vi "visuallyInspectPositionListResults.vi"() -> ()   [LabVIEW 2016]
uses:
  <vilib>/vision/driver/NI_Vision_Acquisition_Software.lvlib
  <vilib>/vision/NI_Vision_Development_Module.lvlib
  <vilib>/regexp/Match Regular Expression.xnode
  <vilib>/Utility/file.llb/Write Delimited Spreadsheet (DBL).vi
panel:
  in  "Gain":dbl(slide)=4.875739644970414 scale=0.0..20.0
  in  "Nloops":i32=1
  in  "OK Button - Dump":bool
  in  "Path to save collected images":path=path "E:/BNL/XYZstage+Camera_CollectedImages/01-31-2017/Images"
  in  "OK Button - Save":bool
  out "Finished!":bool
  out "Image #":i32=79
  out "Error report":errorcluster
  out "Most recently collected image":T1(plugin-control)
  out "XYZ Stage Current Position":T2={"X [-750, 750 mm]"=-61.75289519379574, "Y [-150, 30 mm]"=-124.53559346701012, "Z [-50, 50 mm]"=-0.8115271662620002}
  in  "Axes Speeds [mm/s]":T3={"X Speed"=25.0, "Y Speed"=10.0, "Z Speed"=10.0}
  out "Moving":bool
  in  "Camera Name":refnum<k21>="cam0" caption="IMAQdx Session"
  in  "Object Location [mm]":T4={"Go to X"=-61.753, "Go to Y"=-124.535, "Go to Z"=-0.811426}
  in  "error in (no error)":errorcluster
  in  "Set of Coordinates to Process":dbl[][](array[numeric])=[[-61.665, -28.54, 0.0], [-61.66, -29.04, -0.05], [35.36, -28.5689, -0.5], [35.359, -29.07, -0.5], [35.35, -125.048, -1.1309], [35.327, -124.561, -1.165], [-61.7, -125.017, -0.8146], [-61.753, -124.535, -0.811426], [-61.665, -28.54, 0.0], [-61.66, -29.04, -0.05], [35.36, -28.5689, -0.5], [35.359, -29.07, -0.5], [35.35, -125.048, -1.1309], [35.327, -124.561, -1.165], [-61.7, -125.017, -0.8146], [-61.753, -124.535, -0.811426], [-61.665, -28.54, 0.0], [-61.66, -29.04, -0.05], [35.36, -28.5689, -0.5], [35.359, -29.07, -0.5], [35.35, -125.048, -1.1309], [35.327, -124.561, -1.165], [-61.7, -125.017, -0.8146], [-61.753, -124.535, -0.811426], [-61.665, -28.54, 0.0], [-61.66, -29.04, -0.05], [35.36, -28.5689, -0.5], [35.359, -29.07, -0.5], [35.35, -125.048, -1.1309], [35.327, -124.561, -1.165], [-61.7, -125.017, -0.8146], [-61.753, -124.535, -0.811426], [-61.665, -28.54, 0.0], [-61.66, -29.04, -0.05], [35.36, -28.5689, -0.5], [35.359, -29.07, -0.5], [35.35, -125.048, -1.1309], [35.327, -124.561, -1.165], [-61.7, -125.017, -0.8146], [-61.753, -124.535, -0.811426], [-61.665, -28.54, 0.0], [-61.66, -29.04, -0.05], [35.36, -28.5689, -0.5], [35.359, -29.07, -0.5], [35.35, -125.048, -1.1309], [35.327, -124.561, -1.165], [-61.7, -125.017, -0.8146], [-61.753, -124.535, -0.811426], [-61.665, -28.54, 0.0], [-61.66, -29.04, -0.05], [35.36, -28.5689, -0.5], [35.359, -29.07, -0.5], [35.35, -125.048, -1.1309], [35.327, -124.561, -1.165], [-61.7, -125.017, -0.8146], [-61.753, -124.535, -0.811426], [-61.665, -28.54, 0.0], [-61.66, -29.04, -0.05], [35.36, -28.5689, -0.5], [35.359, -29.07, -0.5], [35.35, -125.048, -1.1309], [35.327, -124.561, -1.165], [-61.7, -125.017, -0.8146], [-61.753, -124.535, -0.811426], [-61.665, -28.54, 0.0], [-61.66, -29.04, -0.05], [35.36, -28.5689, -0.5], [35.359, -29.07, -0.5], [35.35, -125.048, -1.1309], [35.327, -124.561, -1.165], [-61.7, -125.017, -0.8146], [-61.753, -124.535, -0.811426], [-61.665, -28.54, 0.0], [-61.66, -29.04, -0.05], [35.36, -28.5689, -0.5], [35.359, -29.07, -0.5], [35.35, -125.048, -1.1309], [35.327, -124.561, -1.165], [-61.7, -125.017, -0.8146], [-61.753, -124.535, -0.811426]]
  out "Image Array":T1[](array[plugin-control])
  # "Use the index box to specify the image you wish to view"
  # ">>>>"
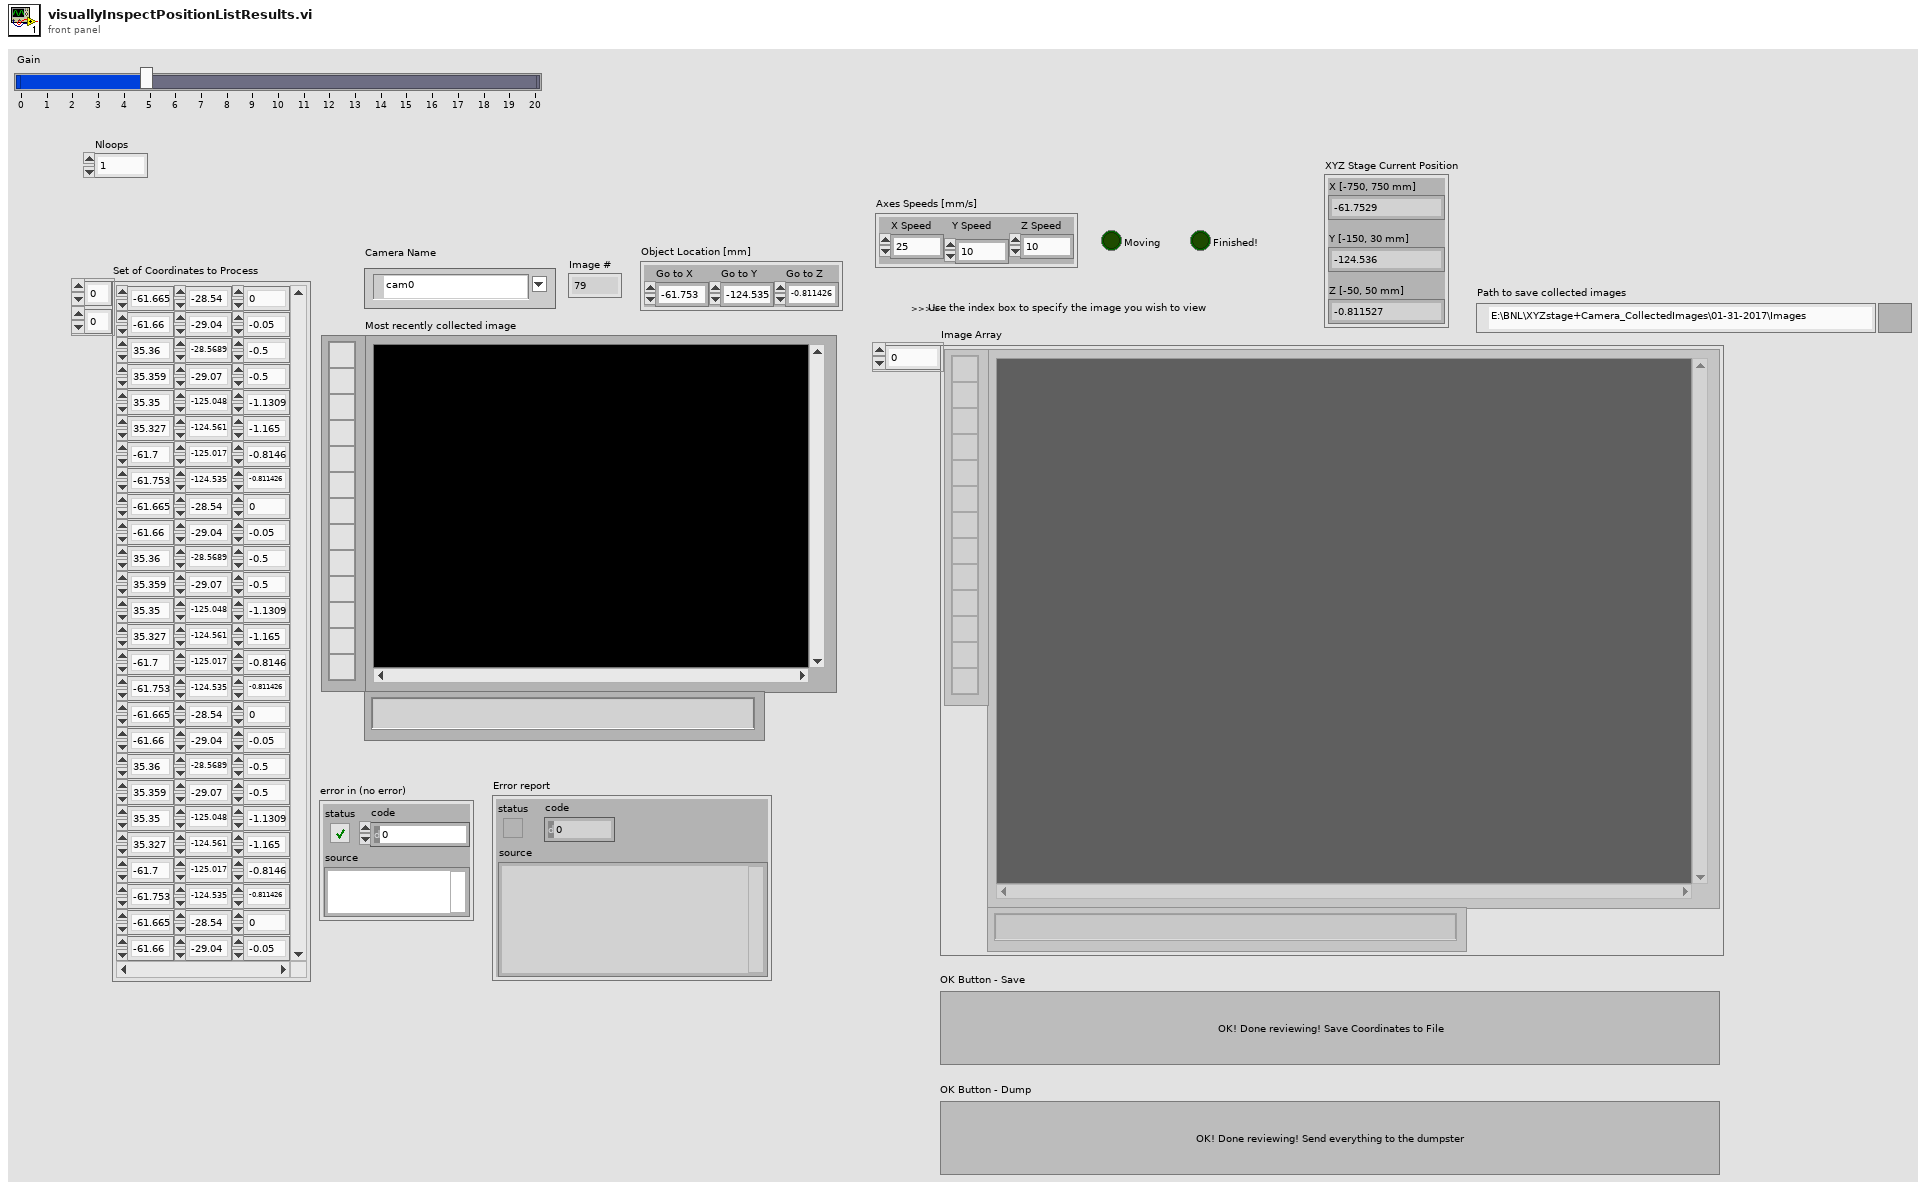
[diagram p1: front panel]
types:
  T1 = typedef "IMAQ Image.ctl" = refnum<image>
  T2 = cluster{"X [-750, 750 mm]":dbl, "Y [-150, 30 mm]":dbl, "Z [-50, 50 mm]":dbl}
  T3 = cluster{"X Speed":dbl, "Y Speed":dbl, "Z Speed":dbl}
  T4 = cluster{"Go to X":dbl, "Go to Y":dbl, "Go to Z":dbl}
  T5 = typedef "IMAQdx.ctl" = refnum<k21>
  T6 = cluster{"Set of Coordinates to Process[0]":dbl, "Set of Coordinates to Process[1]":dbl, "Set of Coordinates to Process[2]":dbl}
  T7 = typedef "Image Type" = u32
  T8 = cluster{"Final X":dbl, "Final Y":dbl, "Final Z":dbl}
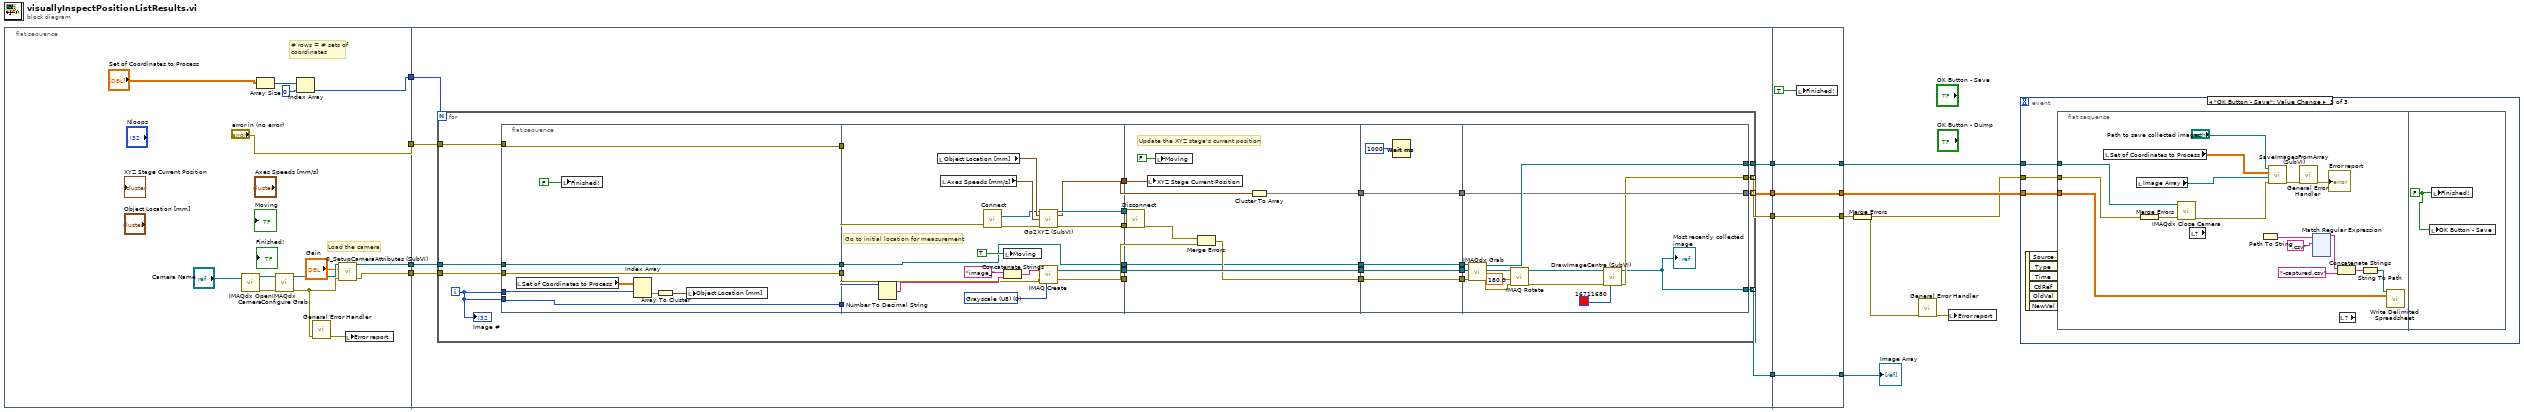
[diagram p0: block diagram]
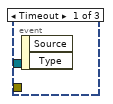
[diagram p2: hidden frame]
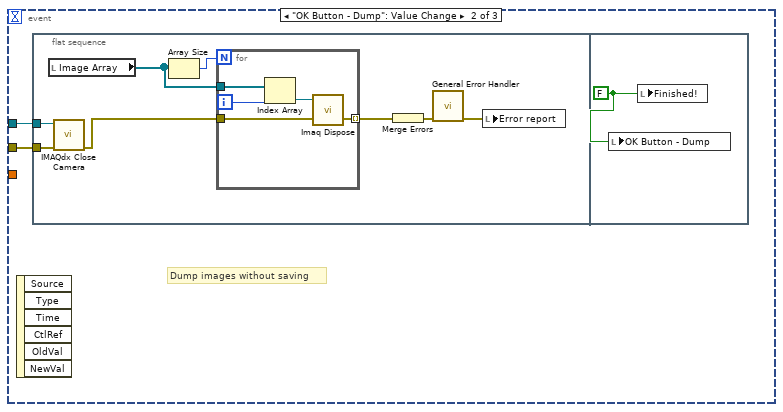
[diagram p3: hidden frame]
diagram:
  n1 = flat-sequence {
    tunnel: [w25] -> w4
    tunnel: ["error in (no error)"] -> w3
    tunnel: [w16] -> w2
    tunnel: [w15] -> w1
    tunnel: [w35] -> w8
    tunnel: [w34] -> w7
    tunnel: [w33] -> w6
    tunnel: [w31] -> w5
    tunnel: w4 -> [w36]
    tunnel: w3 -> [w32]
    tunnel: w2 -> [w30]
    tunnel: w1 -> [w29]
    tunnel: [w119] -> w11
    tunnel: [w120] -> w12
    tunnel: [w121] -> w13
    tunnel: [w122] -> w14
    tunnel: w8 -> [w122]
    tunnel: w7 -> [w121]
    tunnel: w6 -> [w120]
    tunnel: w5 -> [w119]
    frame #0 {
      # "Load the camera"
      # "# rows = # sets of\ncoordinates"
      n2 = call <vilib>:"IMAQdx Open Camera.vi"("Session In"="Camera Name") -> ("error out"=w18:errorcluster, "Session Out"=w17:T5)  [unwired: 2 in, 7 out]
      n3 = Array Size(array="Set of Coordinates to Process") -> (size(s)=w26:i32[])
      n4 = call <vilib>:"IMAQdx Configure Grab.vi"("error in"=w18, "Session In"=w17) -> ("error out"=w22:errorcluster, "Session Out"=w23:T5)  [unwired: 8 out]
      n5 = Index Array(array=w26, index=0) -> (element=w25:i32)
      n6 = call <vilib>:"General Error Handler.vi"("error in (no error)"=w22) -> ("error out"=w20:errorcluster)  [unwired: 2 in, 12 out]
      n7 = call "0_SetupCameraAttributes (SubVI).vi"("error in (no error)"=w22, "Gain"="Gain", "Camera session in"=w23) -> ("error out"=w16:errorcluster, "Camera session out"=w15:T5)  [unwired: 7 in]
      n8 = local write "Error report"(w20) -> ()
    }
    frame #1 {
      n9 = for {
        N: w36 -> [_]
        tunnel: [w54] -> w35 mode=indexing
        tunnel: w32 -> [w52]
        tunnel: w30 -> [w50]
        tunnel: [w46] -> w34
        tunnel: [w45] -> w31 mode=indexing
        tunnel: [w42] -> w33 mode=indexing
        tunnel: w29 -> [w41]
        i -> [w58]
        n10 = flat-sequence {
          tunnel: w58 -> [w68]
          tunnel: w58 -> [w67]
          tunnel: [w67] -> w59
          tunnel: [w66] -> w53
          tunnel: w52 -> [w66]
          tunnel: [w65] -> w51
          tunnel: w50 -> [w65]
          tunnel: w41 -> [w63]
          tunnel: [w63] -> w40
          tunnel: [w83] -> w62
          tunnel: [w82] -> w61
          tunnel: [w81] -> w60
          tunnel: w59 -> [w77]
          tunnel: [w78] -> w55
          tunnel: w53 -> [w75]
          tunnel: w51 -> [w74]
          tunnel: [w73] -> w47
          tunnel: w40 -> [w72]
          tunnel: [w72] -> w39
          tunnel: w62 -> [w98]
          tunnel: w61 -> [w92]
          tunnel: w60 -> [w97]
          tunnel: [w96] -> w56
          tunnel: w55 -> [w96]
          tunnel: [w93] -> w48
          tunnel: w47 -> [w94]
          tunnel: [w91] -> w44
          tunnel: w39 -> [w90]
          tunnel: [w90] -> w37
          tunnel: [w103] -> w57
          tunnel: w56 -> [w103]
          tunnel: [w102] -> w49
          tunnel: w48 -> [w102]
          tunnel: w44 -> [w101]
          tunnel: [w101] -> w43
          tunnel: [w100] -> w38
          tunnel: w37 -> [w100]
          tunnel: w57 -> [w117]
          tunnel: [w107] -> w54
          tunnel: w49 -> [w114]
          tunnel: [w112] -> w46
          tunnel: [w108] -> w45
          tunnel: w43 -> [w111]
          tunnel: [w111] -> w42
          tunnel: w38 -> [w105]
          frame #0 {
            n11 = local read "Set of Coordinates to Process"() -> (w69:dbl[][])
            n12 = local write "Finished!"(FALSE ("Finished!")) -> ()
            n13 = Index Array(array=w69, index (row)=w68) -> (element=w70:dbl[])  [unwired: 1 in]
            n14 = Array To Cluster(array=w70) -> (cluster=w71:T6)
            n15 = local write "Object Location [mm]"(w71) -> ()
          }
          frame #1 {
            w89 = T7 0 items=["Grayscale (U8)", "Grayscale (I16)", "Grayscale (SGL)", "Complex (CSG)", "RGB (U32)", "HSL (U32)", "RGB (U64)", "Grayscale (U16)"] ("Image Type")
            # "Go to initial location for measurement"
            n16 = Number To Decimal String(number=w77) -> (decimal integer string=w76:string)  [unwired: 1 in]
            n17 = local read "Object Location [mm]"() -> (w86:T4)
            n18 = local read "Axes Speeds [mm/s]"() -> (w87:T3)
            n19 = call "Connect.vi"("error in (no error)"=w75) -> ("error out"=w84:errorcluster, "controller"=w85:refnum<k24>)  [unwired: 9 in]
            n20 = local write "Moving"(TRUE ("Moving")) -> ()
            n21 = Concatenate Strings("image_" ("Image Name"), w76) -> (w79:string)
            n22 = call "Go2XYZ (SubVI).vi"(".NET Refnum in"=w85, "Go to Coordinates"=w86, "Axis Speeds"=w87, "error in (no error)"=w84) -> (".NET Refnum out"=w83:refnum<k24>, "Final Position"=w82:T8, "error out"=w81:errorcluster)  [unwired: 7 in, 2 out]
            n23 = call "IMAQ Create"("Image Name"=w79, "Image Type"=w89, "error in (no error)"=w74) -> ("New Image"=w78:T1, "error out"=w73:errorcluster)  [unwired: 1 in, 1 out]
          }
          frame #2 {
            # "Update the XYZ stage's current position"
            n24 = call "Disconnect.vi"("error in (no error)"=w97, "controller"=w98) -> ("error out"=w95:errorcluster)  [unwired: 9 in]
            n25 = local write "XYZ Stage Current Position"(w92) -> ()
            n26 = local write "Moving"(FALSE ("Moving")) -> ()
            n27 = Merge Errors(w95, w94) -> (w93:errorcluster)
            n28 = Cluster To Array(cluster=w92) -> (array=w91:dbl[])
          }
          frame #3 {
            n29 = Wait (ms)(milliseconds to wait=u32 1000) -> ()  [unwired: 1 out]
          }
          frame #4 {
            n30 = call <vilib>:"IMAQdx Grab.vi"("error in"=w114, "Image In"=w117, "Session In"=w105) -> ("error out"=w113:errorcluster, "Image Out"=w116:T1, "Session Out"=w112:T5)  [unwired: 1 in, 5 out]
            n31 = call "IMAQ Rotate"("error in (no error)"=w113, "Angle (degrees)"=sgl 180.0, "Image Src"=w116) -> ("error out"=w109:errorcluster, "Image Dst Out"=w110:T1)  [unwired: 7 in]
            n32 = call "DrawImageCentre (SubVI).vi"("Axis colour"=u32 16711680, "error in (no error)"=w109, "Refnum in"=w110) -> ("error out"=w108:errorcluster, "Refnum out"=w107:T1)  [unwired: 7 in]
            "Most recently collected image" <- w107
          }
        }
        "Image #" <- w58
      }
    }
    frame #2 {
      n33 = local write "Finished!"(TRUE ("Finished!")) -> ()
    }
  }
  n34 = Merge Errors(w11) -> (w9:errorcluster)
  n35 = call <vilib>:"General Error Handler.vi"("error in (no error)"=w9) -> ("error out"=w10:errorcluster)  [unwired: 2 in, 12 out]
  n36 = local write "Error report"(w10) -> ()
  n37 = event shown="[2] \"OK Button - Save\": Value Change" {
    selector: _ -> [_ _ _]
    dyn-events: _ -> [_ _ _]
    timeout: _ -> [_ _ _]
    tunnel: w9 -> [_ w123 w141]
    tunnel: w13 -> [_ w124 w140]
    tunnel: w12 -> [_ _ w139]
    event Timeout {
      n38 = event-data() -> ()  [unwired: 1 in, 2 out]
    }
    event "OK Button - Dump": Value Change {
      # "Dump images without saving"
      n39 = event-data() -> ()  [unwired: 1 in, 6 out]
      n40 = flat-sequence {
        tunnel: w124 -> [w132]
        tunnel: w123 -> [w131]
        frame #0 {
          n41 = local read "Image Array"() -> (w130:T1[])
          n42 = call <vilib>:"IMAQdx Close Camera.vi"("error in"=w131, "Session In"=w132) -> ("error out"=w127:errorcluster)  [unwired: 9 out]
          n43 = Array Size(array=w130) -> (size(s)=w129:i32)
          n44 = for {
            N: w129 -> [_]
            tunnel: w130 -> [w137]
            tunnel: w127 -> [w134]
            tunnel: [w133] -> w126 mode=indexing
            i -> [w136]
            n45 = Index Array(array=w137, index=w136) -> (element=w135:T1)
            n46 = call "Imaq Dispose"("Image"=w135, "error in (no error)"=w134) -> ("error out"=w133:errorcluster)  [unwired: 4 in]
          }
          n47 = Merge Errors(w126) -> (w125:errorcluster)
          n48 = call <vilib>:"General Error Handler.vi"("error in (no error)"=w125) -> ("error out"=w128:errorcluster)  [unwired: 2 in, 12 out]
          n49 = local write "Error report"(w128) -> ()
        }
        frame #1 {
          w138 = FALSE ("Finished!")
          n50 = local write "OK Button - Dump"(w138) -> ()
          n51 = local write "Finished!"(w138) -> ()
        }
      }
    }
    event "OK Button - Save": Value Change {
      n52 = event-data() -> ()  [unwired: 1 in, 6 out]
      n53 = flat-sequence {
        tunnel: w141 -> [w149]
        tunnel: w140 -> [w148]
        tunnel: w139 -> [w147]
        frame #0 {
          n54 = local read "Set of Coordinates to Process"() -> (w142:dbl[][])
          n55 = local read "Image Array"() -> (w146:T1[])
          n56 = Merge Errors(w149) -> (w150:errorcluster)
          n57 = call <vilib>:"IMAQdx Close Camera.vi"("error in"=w150, "Session In"=w148) -> ("error out"=w145:errorcluster)  [unwired: 9 out]
          n58 = local read item#-1() -> ()  [unwired: 1 out]
          n59 = Path To String() -> (string=w152:string)  [unwired: 1 in]
          n60 = call "SaveImagesFromArray (SubVI).vi"("error in (no error)"=w145, "Array of Images"=w146, "XY Camera Coordinates"=w142, "Path to save collected images"="Path to save collected images") -> ("error out"=w144:errorcluster)  [unwired: 7 in]
          n61 = call <vilib>:"General Error Handler.vi"("error in (no error)"=w144) -> ("error out"=→"Error report":errorcluster)  [unwired: 2 in, 12 out]
          n62 = xnode "Match Regular Expression"("input string"=w152, "regular expression"=".csv") -> ("before match"=w155:string)  [unwired: 4 in, 4 out]
          n63 = Concatenate Strings(w155, "-captured.csv" ("name or relative path")) -> (w156:string)
          n64 = local read item#-1() -> ()  [unwired: 1 out]
          n65 = String To Path(string=w156) -> (path=w157:path)
          n66 = call-poly <vilib>:"Write Delimited Spreadsheet.vi"("file path (dialog if empty)"=w157, "2D data"=w147) -> ()  [unwired: 12 in, 2 out]
        }
        frame #1 {
          w272 = FALSE ("Finished!")
          n67 = local write "OK Button - Save"(w272) -> ()
          n68 = local write "Finished!"(w272) -> ()
        }
      }
    }
  }
  "Image Array" <- w14
